vi "Datatype Assert.vi"(8 "error in (no error)":errorcluster, 10 "Data Type":variant, 11 "JSON":string) -> (0 "error out":errorcluster, 1 "error out (Assert)":errorcluster, 2 "JSONText (Assert)":string, 3 "JKIJSON (Assert)":string)   [LabVIEW 2018, in "JSON to LVConstant Test.lvlib"]
uses:
  JSON to LVConstant Test.lvlib
  <vilib>/Utility/miscctls.llb/LVPointTypeDef.ctl
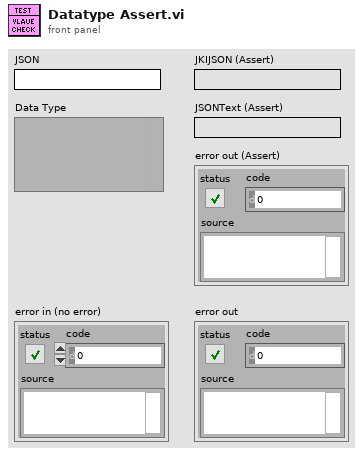
[diagram p1: front panel]
types:
  T1 = enum8{"Probe", "Diagram", "Panel Control", "3D Panel Control", "Dialog Panel Control", "Panel Indicator", "3D Panel Indicator", "Dialog Panel Indicator", "Power PC Control", "Power PC Indicator", "Silver Control", "Silver Indicator", "NXG Style Control", "NXG Style Indicator"}
  T2 = typedef "LVPointTypeDef.ctl" = cluster{"Horizontal":i16, "Vertical":i16}
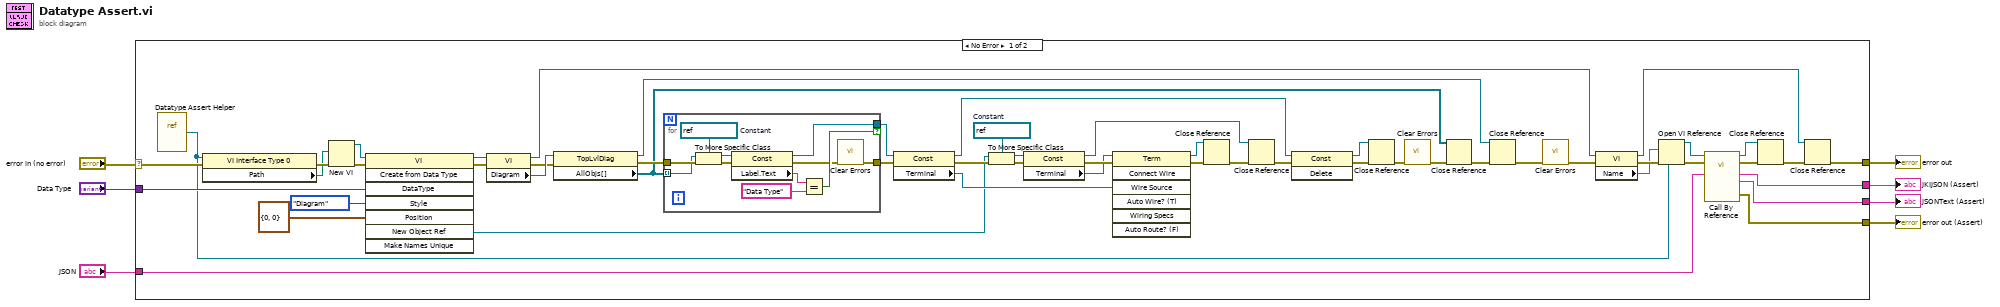
[diagram p0: block diagram]
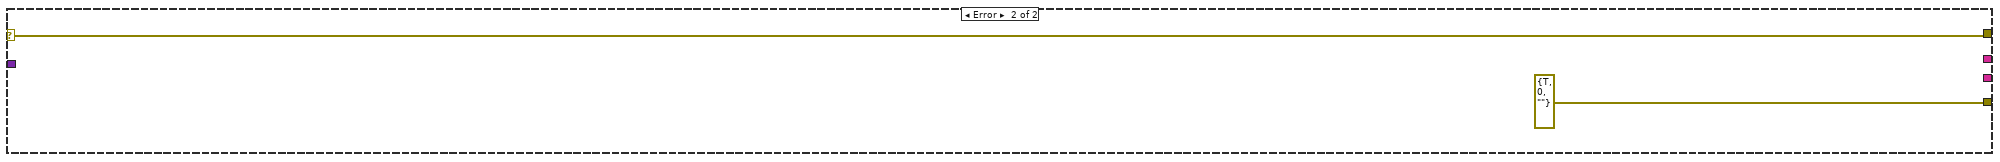
[diagram p2: hidden frame]
diagram:
  n1 = case shown="No Error" "error in (no error)" {
    selector: "error in (no error)" -> [w13 w73]
    tunnel: "JSON" -> [w20 _]
    tunnel: [w19 _] -> w2
    tunnel: [w18 errorcluster {"status"=TRUE, "code"=0, "source"=""} ("error out")] -> w6
    tunnel: [w14 w73] -> w5
    tunnel: "Data Type" -> [w12 _]
    tunnel: [w10 _] -> w1
    frame No Error {
      w50 = refnum<vi> refnum  # Constant
      n2 = vi-ref "Datatype Assert Helper.vi"() -> (w11:refnum<vi>)
      n3 = property class="VI Interface Type 0"(reference=w11, error in=w13) -> (error out=w54:errorcluster, "Path"=w28:path)  [unwired: 1 out]
      n4 = New VI(8:w54, 10:w28) -> (0:w55:errorcluster, 3:w8:refnum<vi>)  [unwired: 5 in]
      n5 = invoke class="VI" method="Create from Data Type"(reference=w8, error in=w55, "DataType"=w12, "Style"=T1."Diagram", "Position"=T2 {"Horizontal"=0, "Vertical"=0}) -> (reference out=w37:refnum<vi>, error out=w38:errorcluster, "New Object Ref"=w40:refnum<vi>)  [unwired: 3 in, 5 out]
      n6 = property class="VI"(reference=w37, error in=w38) -> (reference out=w24:refnum<vi>, error out=w39:errorcluster, "Diagram"=w45:refnum<vi>)
      n7 = property class="TopLvlDiag"(reference=w45, error in=w39) -> (reference out=w53:refnum<vi>, error out=w60:errorcluster, "AllObjs[]"=w57:refnum<vi>[])
      n8 = for {
        tunnel: w57 -> [w64] mode=indexing
        tunnel: [w69] -> w58 if=w68
        tunnel: w60 -> [w71]
        tunnel: [w61] -> w59
        w62 = refnum<vi> refnum  # Constant
        n9 = To More Specific Class(target class=w62, reference=w64, error in=w71) -> (specific class reference=w63:refnum<vi>, error out=w65:errorcluster)
        n10 = property class="Const"(reference=w63, error in=w65) -> (reference out=w69:refnum<vi>, error out=w67:errorcluster, "Label.Text"=w66:string)
        n11 = Equal?(x=w66, y="Data Type") -> (x = y?=w68:bool)
        n12 = call <vilib>:"Clear Errors.vi"("error in (no error)"=w67) -> ("error out"=w61:errorcluster)  [unwired: 5 in, 1 out]
      }
      n13 = property class="Const"(reference=w58, error in=w59) -> (reference out=w41:refnum<vi>, error out=w56:errorcluster, "Terminal"=w46:refnum<vi>)
      n14 = To More Specific Class(target class=w50, reference=w40, error in=w56) -> (specific class reference=w51:refnum<vi>, error out=w52:errorcluster)
      n15 = property class="Const"(reference=w51, error in=w52) -> (reference out=w47:refnum<vi>, error out=w49:errorcluster, "Terminal"=w48:refnum<vi>)
      n16 = invoke class="Term" method="Connect Wire"(reference=w48, error in=w49, "Wire Source"=w46) -> (reference out=w36:refnum<vi>, error out=w42:errorcluster)  [unwired: 4 in, 5 out]
      n17 = Close Reference(reference=w36, error in (no error)=w42) -> (error out=w35:errorcluster)
      n18 = Close Reference(reference=w47, error in (no error)=w35) -> (error out=w34:errorcluster)
      n19 = invoke class="Const" method="Delete"(reference=w41, error in=w34) -> (reference out=w32:refnum<vi>, error out=w33:errorcluster)  [unwired: 1 in, 1 out]
      n20 = Close Reference(reference=w32, error in (no error)=w33) -> (error out=w31:errorcluster)
      n21 = call <vilib>:"Clear Errors.vi"("error in (no error)"=w31) -> ("error out"=w30:errorcluster)  [unwired: 5 in, 1 out]
      n22 = Close Reference(reference=w57, error in (no error)=w30) -> (error out=w29:errorcluster)
      n23 = Close Reference(reference=w53, error in (no error)=w29) -> (error out=w27:errorcluster)
      n24 = call <vilib>:"Clear Errors.vi"("error in (no error)"=w27) -> ("error out"=w9:errorcluster)  [unwired: 5 in, 1 out]
      n25 = property class="VI"(reference=w24, error in=w9) -> (reference out=w22:refnum<vi>, error out=w25:errorcluster, "Name"=w23:string)
      n26 = Open VI Reference(type specifier VI Refnum (for type only)=w11, vi path=w23, error in (no error)=w25) -> (vi reference=w21:refnum<vi>, error out=w26:errorcluster)  [unwired: 3 in]
      n27 = call-by-ref "?"(reference=w21, error in=w26, "JSON"=w20) -> (reference out=w17:refnum<vi>, error out=w16:errorcluster, 0:"error out"=w18:errorcluster, "JSONText (Assert)"=w10:string, "JKIJSON (Assert)"=w19:string)  [unwired: 8 in]
      n28 = Close Reference(reference=w17, error in (no error)=w16) -> (error out=w15:errorcluster)
      n29 = Close Reference(reference=w22, error in (no error)=w15) -> (error out=w14:errorcluster)
    }
    frame Error {
    }
  }
  "error out" <- w5
  "error out (Assert)" <- w6
  "JKIJSON (Assert)" <- w2
  "JSONText (Assert)" <- w1
